vi "Get Attribute I32.vi"(8 "error in":errorcluster, 10 "Attribute":string, 11 "Config from EXCEL in":refnum<class "Config from EXCEL.lvclass">) -> (0 "error out":errorcluster, 2 "Value":i32, 3 "Config from EXCEL out":refnum<class "Config from EXCEL.lvclass">)   [LabVIEW 2025, in "Config from EXCEL.lvclass"]
uses:
  Config from EXCEL.lvclass
  Config from EXCEL.lvclass/Config from EXCEL.ctl
  Open-Xml-LabVIEW/Source/Open Xml.lvlib
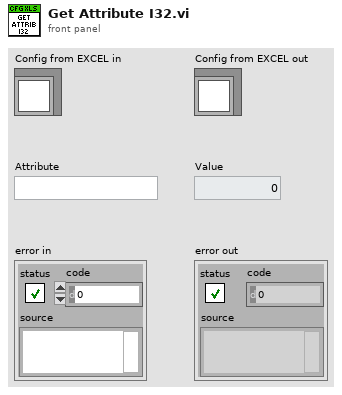
[diagram p1: front panel]
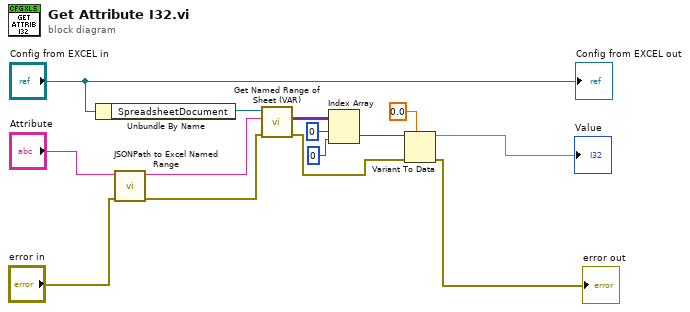
[diagram p0: block diagram]
diagram:
  n1 = Unbundle By Name("Config from EXCEL in") -> ("SpreadsheetDocument"=w14:refnum<k24>)
  n2 = call "JSONPath to Excel Named Range.vi"("error in"="error in", "JSONPath"="Attribute") -> ("error out"=w9:errorcluster, "Named Range"=w13:string)  [unwired: 8 in]
  n3 = call "Get Named Range of Sheet (VAR).vi"("error in"=w9, "Named Range Identifier"=w13, "SpreadsheetDocument"=w14) -> ("error out"=w2:errorcluster, "Cells"=w12:variant[][])  [unwired: 6 in, 1 out]
  n4 = Index Array(array=w12, index (row)=0, index (col)=0) -> (element=w5:variant)
  n5 = Variant To Data(error in=w2, type=0.0, Variant=w5) -> (data=→"Value":dbl, error out=→"error out":errorcluster)
  "Config from EXCEL out" <- "Config from EXCEL in"
